vi "read_params.vi"(8 "error in (no error)":errorcluster, 11 "IsotonicRegression in":refnum<class "IsotonicRegression.lvclass">) -> (0 "error out":errorcluster, 2 "params":T1={"y_min"={"y_min_type"="None", "y_min_float"=0.0}, "y_max"={"y_max_type"="None", "y_max_float"=0.0}, "increasing"={"increasing_type"="bool", "increasing_bool"=TRUE}, "out_of_bounds"="nan"}, 3 "IsotonicRegression out":refnum<class "IsotonicRegression.lvclass">)   [LabVIEW 2020, in "IsotonicRegression.lvclass"]
uses:
  IsotonicRegression.lvclass
  Controls/isotonic_regression_params.ctl
  IsotonicRegression.lvclass/IsotonicRegression.ctl
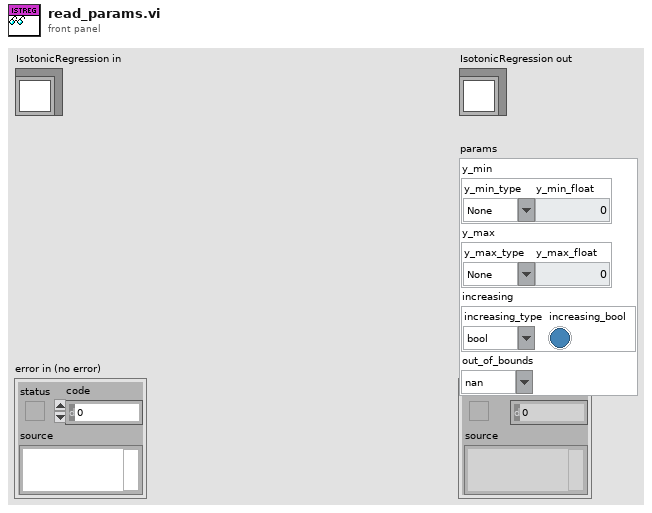
[diagram p1: front panel]
types:
  T1 = typedef "isotonic_regression_params.ctl" = cluster{"y_min":cluster{"y_min_type":string, "y_min_float":dbl}, "y_max":cluster{"y_max_type":string, "y_max_float":dbl}, "increasing":cluster{"increasing_type":string, "increasing_bool":bool}, "out_of_bounds":string}
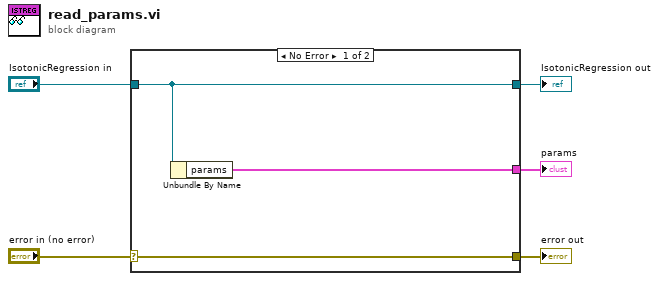
[diagram p0: block diagram]
diagram:
  n1 = case shown="No Error" "error in (no error)" {
    selector: "error in (no error)" -> [w8 w9]
    tunnel: [w8 w9] -> w4
    tunnel: [w7 w10] -> w2
    tunnel: "IsotonicRegression in" -> [w7 w10]
    tunnel: [w6 _] -> w1
    frame No Error {
      n2 = Unbundle By Name(w7) -> ("params"=w6:T1)
    }
    frame Error {
    }
  }
  "error out" <- w4
  "IsotonicRegression out" <- w2
  "params" <- w1
